vi "Send Event.vi"(0 "StatD Interface in":refnum<class "StatD Interface.lvclass">, 1 "Tags":string[](array[string]), 3 "Tag Values":string[](array[string]), 5 "Event Title":string, 7 "Event Text":string, 9 "Event Type (info)":T2=enum."info", 11 "error in (no error)":errorcluster, 12 "Priority (normal)":T1=enum."normal", 13 "Aggregation Key (none)":string) -> (4 "StatD Interface out":refnum<class "StatD Interface.lvclass">, 15 "error out":errorcluster)   [LabVIEW 2011, in "StatD Interface.lvclass"]
doc: "Sends an event to the statd collector."
uses:
  StatD Interface.lvclass
  Controls/Event Types.ctl
  Controls/Priorities.ctl
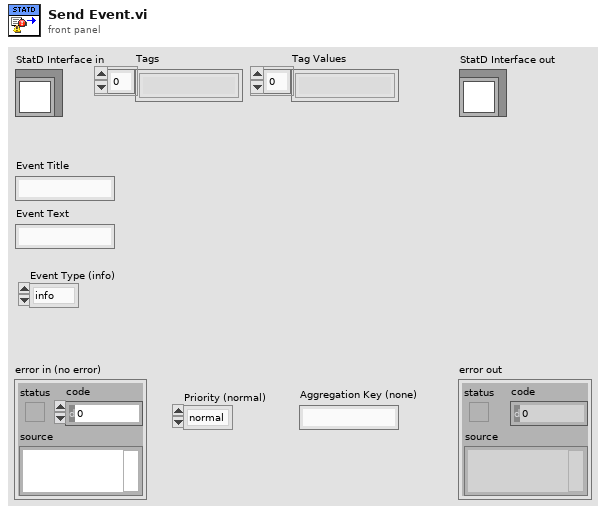
[diagram p1: front panel]
types:
  T1 = typedef "StatD Interface.lvclass/Priorities.ctl" = enum16{"low", "normal"}
  T2 = typedef "StatD Interface.lvclass/Event Types.ctl" = enum16{"error", "warning", "info", "success"}
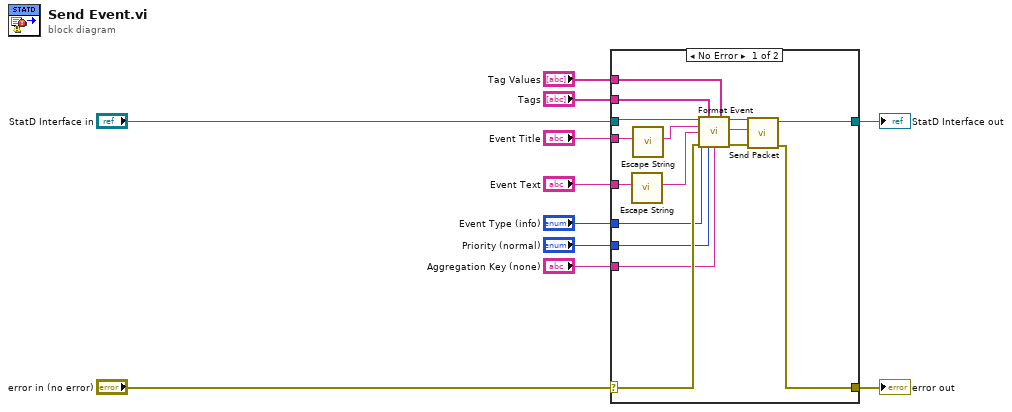
[diagram p0: block diagram]
diagram:
  n1 = case shown="No Error" "error in (no error)" {
    selector: "error in (no error)" -> [w21 w29]
    tunnel: [w24 w29] -> w10
    tunnel: [w25 w28] -> w8
    tunnel: "StatD Interface in" -> [w23 w28]
    tunnel: "Tags" -> [w20 _]
    tunnel: "Tag Values" -> [w19 _]
    tunnel: "Event Title" -> [w18 _]
    tunnel: "Event Text" -> [w17 _]
    tunnel: "Event Type (info)" -> [w16 _]
    tunnel: "Priority (normal)" -> [w15 _]
    tunnel: "Aggregation Key (none)" -> [w14 _]
    frame No Error {
      n2 = call <vilib>:"Escape String.vi"("Message In"=w17) -> ("Message Out"=w12:string)  [unwired: 10 in]
      n3 = call <vilib>:"Escape String.vi"("Message In"=w18) -> ("Message Out"=w13:string)  [unwired: 10 in]
      n4 = call "Format Event.vi"("StatD Interface in"=w23, "Tags"=w20, "Tag Values"=w19, "Event Title"=w13, "Event Text"=w12, "Event Type"=w16, "error in (no error)"=w21, "Priority (normal)"=w15, "Aggregation Key (none)"=w14) -> ("StatD Interface out"=w27:refnum<class "StatD Interface.lvclass">, "Packet"=w26:string, "error out"=w22:errorcluster)  [unwired: 4 in]
      n5 = call "Send Packet.vi"("error in (no error)"=w22, "Packet"=w26, "StatD Interface in"=w27) -> ("error out"=w24:errorcluster, "StatD Interface out"=w25:refnum<class "StatD Interface.lvclass">)  [unwired: 7 in]
    }
    frame Error {
    }
  }
  "error out" <- w10
  "StatD Interface out" <- w8
